vi "Handle TCP Connection.vi"(4 "Remote Port":u16, 6 "Remote Host":string, 7 "TCPMessageAPI":refnum<class "TCPMessageAPI.lvclass">, 8 "error in (no error)":errorcluster, 9 "Node ID":u32, 10 "Connection State":T1, 11 "Simple TCP Handler in":refnum<class "Simple TCP Handler.lvclass">) -> (0 "error out":errorcluster, 3 "Simple TCP Handler out":refnum<class "Simple TCP Handler.lvclass">)   [LabVIEW 2020, in "VectoScratch.lvlib" / "Simple TCP Handler.lvclass"]
uses:
  Simple TCP Handler.lvclass
  Vecto/Connection State.ctl
  Vecto/TCPMessageService/TCPMessageAPI.lvclass
  Simple TCP Handler.lvclass/Simple TCP Handler.ctl
  Vecto/Vecto.lvlib
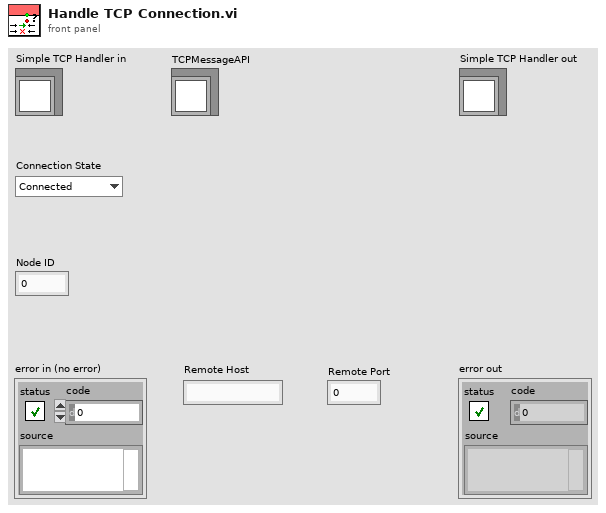
[diagram p1: front panel]
types:
  T1 = typedef "Vecto.lvlib/Connection State.ctl" = enum16{"Connected", "Disconnected"}
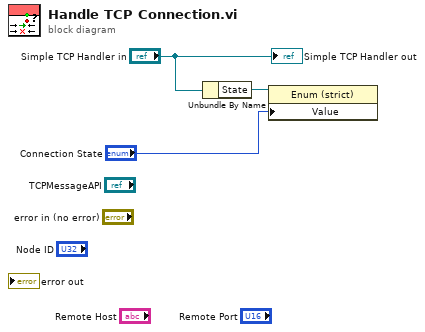
[diagram p0: block diagram]
diagram:
  n1 = Unbundle By Name("Simple TCP Handler in") -> ("State"=w2:refnum<vi>)
  n2 = property class="Enum (strict)"(reference=w2, "Value"="Connection State") -> ()  [unwired: 1 in, 2 out]
  "Simple TCP Handler out" <- "Simple TCP Handler in"
